vi "Apply Tombstone Target.vi"   [LabVIEW 2018, in "Tests.lvlib" / "Toolkit.lvlib" / "Unit.lvlib"]
uses:
  Unit.lvlib
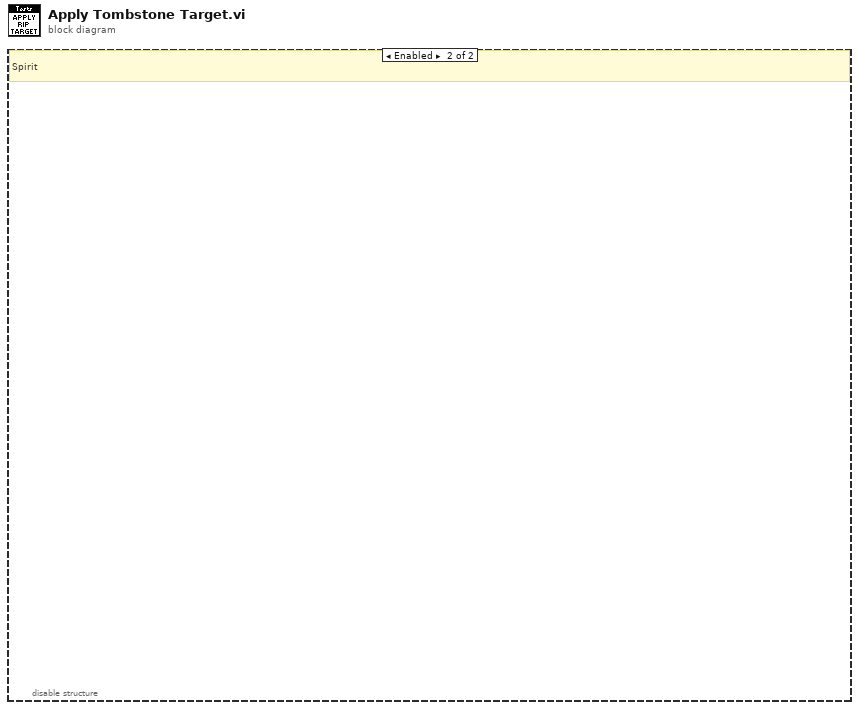
[diagram p0: block diagram]
diagram:
  n1 = disable-structure shown="Enabled" {
    frame Disabled {
      # "Corpse"
    }
    frame Enabled {
      # "Spirit"
    }
  }
